vi "blocktemplate.vi"(4 "Block Size (20)":u32=20, 8 "Piece Array":i16[][](array[numeric]), 10 "board array":i16[][](array[numeric]), 11 "color array":u32[](array[colorbox])=[0, 15790080, 8388608, 8421376, 128, 32896, 8388736, 32896]) -> (3 "Picture":picture)   [LabVIEW 2018]
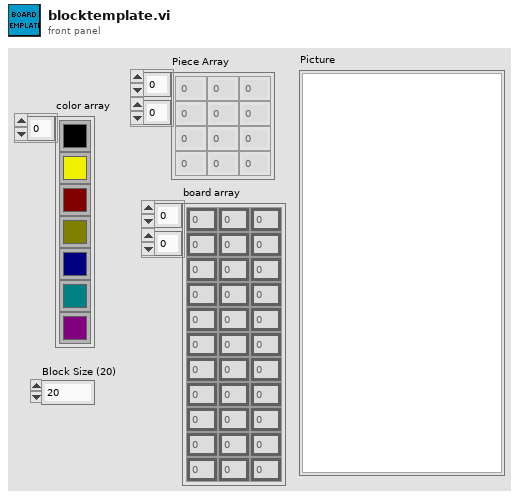
[diagram p1: front panel]
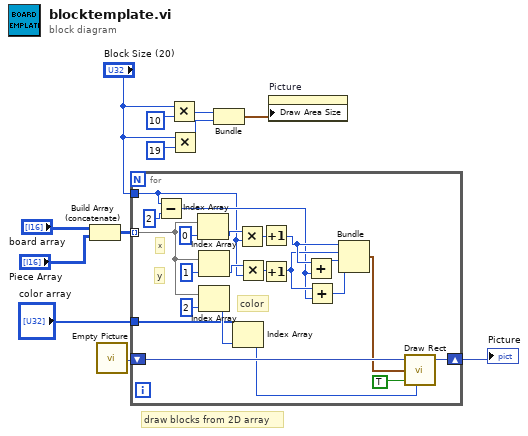
[diagram p0: block diagram]
diagram:
  # "draw blocks from 2D array"
  n1 = Build Array (concatenate)("board array", "Piece Array") -> (w9:i16[][])
  n2 = call "Empty Picture"() -> ("empty picture"=w2:picture)
  n3 = for {
    shift-right: [w21] -> w1
    shift-left: w2 -> [w22]
    tunnel: w9 -> [w31] mode=indexing
    tunnel: "Block Size (20)" -> [w13]
    tunnel: "color array" -> [w29]
    # "y"
    # "x"
    # "color"
    n4 = Subtract(x=w13, y=u32 2) -> (x-y=w25:u32)
    n5 = Index Array(array=w31, index=0) -> (element=w17:i16)
    n6 = Index Array(array=w31, index=1) -> (element=w16:i16)
    n7 = Index Array(array=w31, index=2) -> (element=w30:i16)
    n8 = Index Array(array=w29, index=w30) -> (element=w18:u32)
    n9 = Multiply(x=w17, y=w13) -> (x*y=w14:u32)
    n10 = Multiply(x=w16, y=w13) -> (x*y=w15:u32)
    n11 = Increment(x=w14) -> (x+1=w27:u32)
    n12 = Increment(x=w15) -> (x+1=w26:u32)
    n13 = Add(x=w27, y=w25) -> (x+y=w24:u32)
    n14 = Add(x=w26, y=w25) -> (x+y=w23:u32)
    n15 = Bundle(w27, w26, w24, w23) -> (w20:cluster{u32, u32, u32, u32})  [unwired: 1 in]
    n16 = call <vilib>:"Draw Rect.vi"("picture"=w22, "rect"=w20, "fill?(F)"=TRUE, "color(black)"=w18) -> ("new picture"=w21:picture)  [unwired: 5 in]
  }
  "Picture" <- w1
  n17 = Multiply(x="Block Size (20)", y=u32 10) -> (x*y=w4:u32)
  n18 = Multiply(x="Block Size (20)", y=u32 19) -> (x*y=w3:u32)
  n19 = Bundle(w4, w3) -> (w7:cluster{u32, u32})  [unwired: 1 in]
  n20 = property on="Picture" class="Pict"("Draw Area Size"=w7) -> ()  [unwired: 2 in, 2 out]
